vi "GV framegate.vi"() -> ()   [LabVIEW 2017]
panel:
  out "Framegate":bool
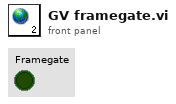
[diagram p1: front panel]
diagram:
